vi "thermometer.vi"(10 "Boolean":bool, 11 "Thermometer F":dbl) -> (3 "Numeric":dbl)   [LabVIEW 2020]
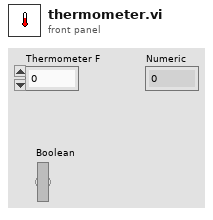
[diagram p1: front panel]
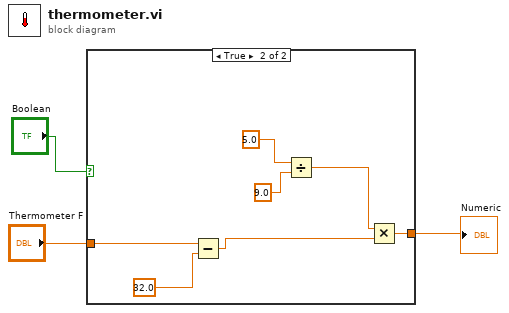
[diagram p0: block diagram]
diagram:
  n1 = case shown="True" "Boolean" {
    tunnel: [w4 w6] -> w3
    tunnel: "Thermometer F" -> [w4 w5]
    frame False {
    }
    frame True {
      n2 = Subtract(x=w5, y=32.0) -> (x-y=w7:dbl)
      n3 = Divide(x=5.0, y=9.0) -> (x/y=w8:dbl)
      n4 = Multiply(x=w8, y=w7) -> (x*y=w6:dbl)
    }
  }
  "Numeric" <- w3
